vi "Get Menu Context ID.vi"(4 "error in (no error)":errorcluster, 6 "Menu Context":T1, 7 "Connection In":refnum<k7>) -> (0 "error out":errorcluster, 2 "context_id":i32, 3 "Connection Out":refnum<k7>)   [LabVIEW 2020, in "Config Data.lvlib" / "Config Data_DB_ADO.lvclass"]
uses:
  Config Data_DB_ADO.lvclass
  toolbox/ADO Database Drivers/ADO Database Drivers.lvlib
  typedefs/Menu Context Selections.ctl
  Config Data.lvclass
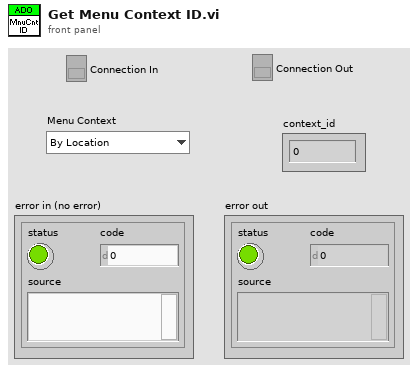
[diagram p1: front panel]
types:
  T1 = typedef "Config Data.lvlib/Config Data.lvclass/Menu Context Selections.ctl" = enum16{"By Location", "By Function"}
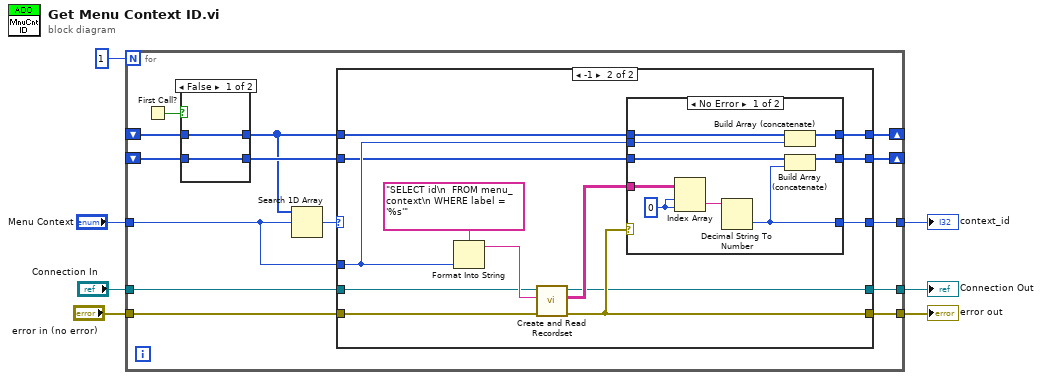
[diagram p0: block diagram]
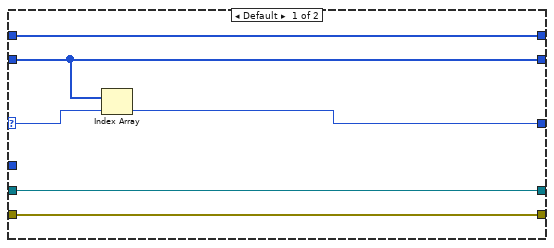
[diagram p3: hidden frame]
diagram:
  n1 = for {
    N: 1 -> [_]
    tunnel: "error in (no error)" -> [w21]
    tunnel: [w20] -> w7
    shift-right: [w19] -> _
    shift-left: _ -> [w15]
    tunnel: "Connection In" -> [w18]
    tunnel: [w17] -> w4
    tunnel: "Menu Context" -> [w9]
    shift-right: [w16] -> _
    shift-left: _ -> [w14]
    tunnel: [w8] -> w3
    n2 = First Call?() -> (First Call?: T/F=w12:bool)
    n3 = case shown="False" w12 {
      tunnel: w15 -> [w23 _]
      tunnel: w14 -> [w22 _]
      tunnel: [w23 _] -> w13
      tunnel: [w22 _] -> w10
      frame False {
      }
      frame True {
      }
    }
    n4 = Search 1D Array(1D array=w10, element=w9) -> (index of element=w11:i32)  [unwired: 1 in]
    n5 = case shown="-1" w11 {
      selector: w11 -> [w26 _]
      tunnel: w21 -> [w29 w36]
      tunnel: [w29 w39] -> w20
      tunnel: w13 -> [w25 w32]
      tunnel: [w25 w31] -> w19
      tunnel: w18 -> [w28 w38]
      tunnel: [w28 w37] -> w17
      tunnel: w9 -> [_ w33]
      tunnel: [w27 w35] -> w16
      tunnel: w10 -> [w27 w34]
      tunnel: [w24 w30] -> w8
      frame Default {
        n6 = Index Array(array=w25, index=w26) -> (element=w24:i32)
      }
      frame -1 {
        n7 = Format Into String(format string="SELECT id\n  FROM menu_context\n WHERE label = '%s'", w33) -> (resulting string=w42:string)  [unwired: 2 in, 1 out]
        n8 = call "Create and Read Recordset.vi"("error in (no error)"=w36, "Source"=w42, "Connection In"=w38) -> ("error out"=w39:errorcluster, "DB Data"=w41:string[][], "Connection Out"=w37:refnum<k7>)  [unwired: 2 in, 2 out]
        n9 = case shown="No Error" w39 {
          tunnel: w41 -> [w51 _]
          tunnel: [w43 _] -> w30
          tunnel: [w46 w53] -> w35
          tunnel: w34 -> [w48 w53]
          tunnel: w33 -> [w47 _]
          tunnel: w32 -> [w45 w52]
          tunnel: [w44 w52] -> w31
          frame No Error {
            w50 = 0 ("disabled index (col)")
            n10 = Index Array(array=w51, index (row)=w50, index (col)=w50) -> (element=w49:string)
            n11 = Decimal String To Number(string=w49) -> (number=w43:i32)  [unwired: 2 in, 1 out]
            n12 = Build Array (concatenate)(w48, w47) -> (w46:T1[])
            n13 = Build Array (concatenate)(w45, w43) -> (w44:i32[])
          }
          frame Error {
          }
        }
      }
    }
  }
  "context_id" <- w3
  "error out" <- w7
  "Connection Out" <- w4
